vi "Apply Material Theme.vi"(8 "error in":errorcluster, 11 "VI Refnum":refnum<vi>) -> (0 "error out":errorcluster)   [LabVIEW 2021]
doc: "Show this VI and let user define a new path/theme to apply to the VI.\n\n->Will be invoked with Quick Drop as a way to easily change the theme quickly during edit mode\n\n<b>Code Developed By:</b>\nTechnology Service Corporation\nwww.tsc.com/atcs\n\nDeveloper:\nDaniel Coons"
uses:
  Material Theme/Material Theme.lvclass
  user32.dll
panel:
  out "Name of VI":string
  in  "Theme":u16(ring) items=["Light", "Light Medium Contrast", "Light High Contrast", "Dark", "Dark Medium Contrast", "Dark High Contrast"]
  in  "done":bool
  out "header":bool
  in  "Path to theme file":path
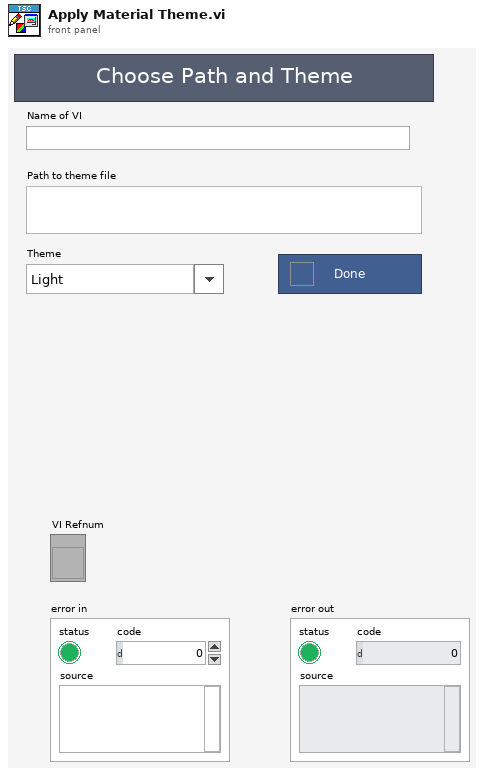
[diagram p1: front panel]
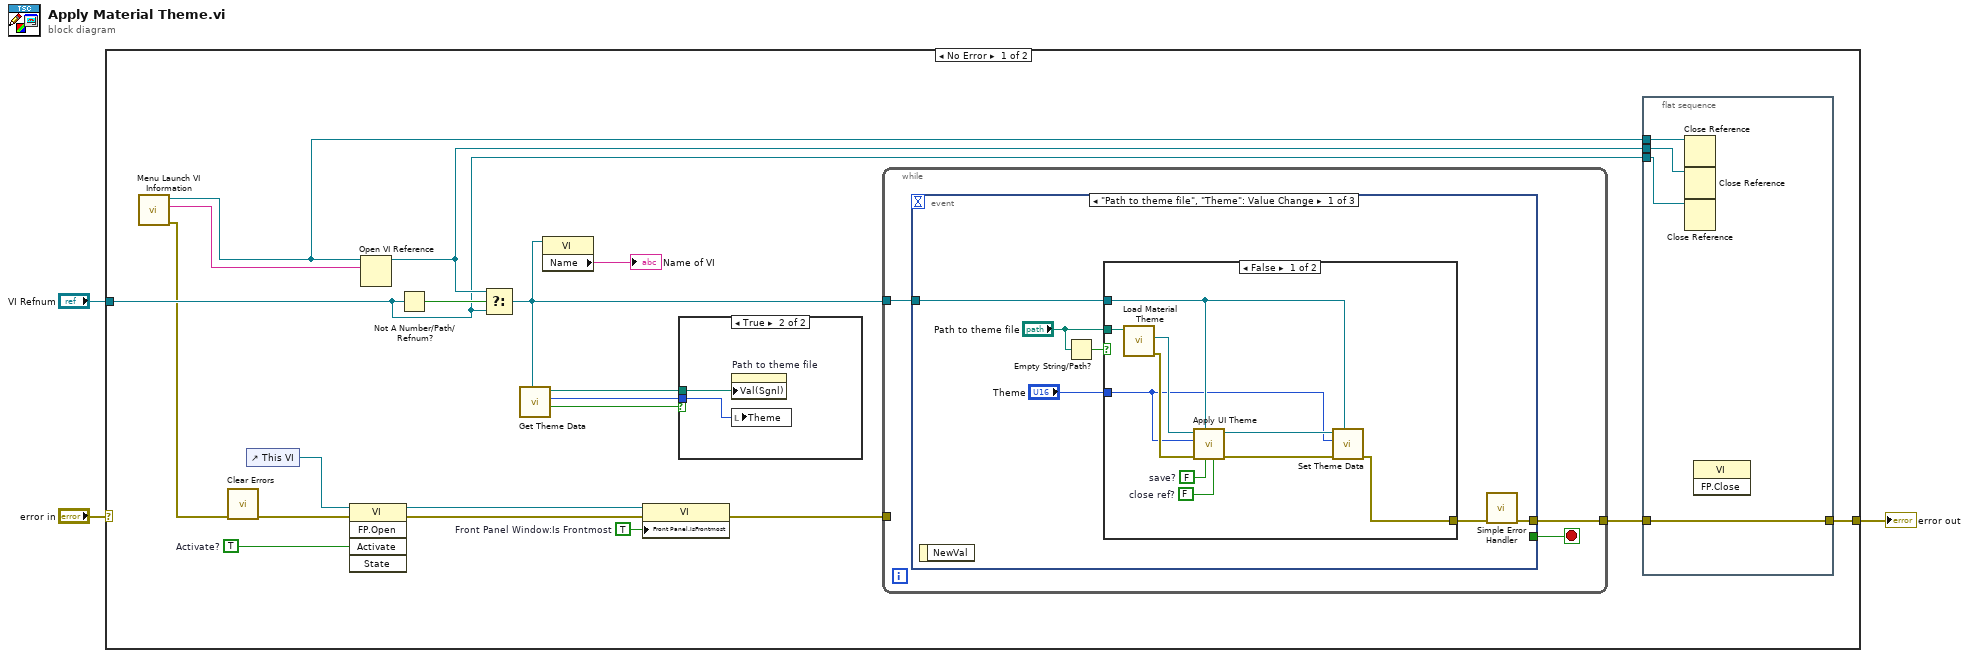
[diagram p0: block diagram]
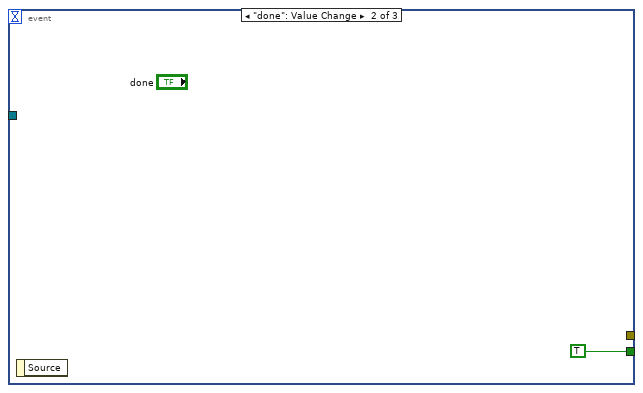
[diagram p4: hidden frame]
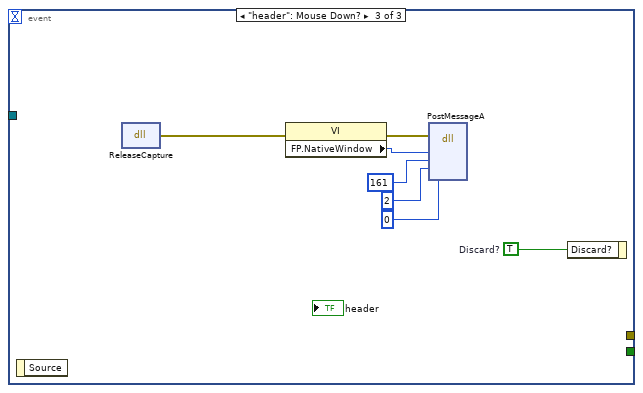
[diagram p5: hidden frame]
diagram:
  n1 = case shown="No Error" "error in" {
    selector: "error in" -> [_ w57]
    tunnel: "VI Refnum" -> [w13 _]
    tunnel: [w20 w57] -> w2
    frame No Error {
      w17 = TRUE  # Front Panel Window:Is Frontmost
      w22 = TRUE  # Activate?
      n2 = call <vilib>:"Menu Launch VI Information.vi"() -> ("error out"=w10:errorcluster, "Menu Launch:VI"=w11:string, "Menu Launch:App"=w12:refnum<vi>)  [unwired: 9 in]
      n3 = call <vilib>:"Clear Errors.vi"("error in (no error)"=w10) -> ("error out"=w8:errorcluster)  [unwired: 5 in, 1 out]
      n4 = control-ref of="This VI"() -> (w9:refnum<vi>)
      n5 = invoke class="VI" method="FP.Open"(reference=w9, error in=w8, "Activate"=w22) -> (reference out=w18:refnum<vi>, error out=w23:errorcluster)  [unwired: 2 in, 3 out]
      n6 = Open VI Reference(application reference (local)=w12, vi path=w11) -> (vi reference=w14:refnum<vi>)  [unwired: 4 in, 1 out]
      n7 = Not A Number/Path/Refnum?(number/path/refnum=w13) -> (NaN/Path/Refnum?=w16:bool)
      n8 = Select(t=w14, s=w16, f=w13) -> (s? t:f=w7:refnum<vi>)
      n9 = call "Get Theme Data.vi"("VI Refnum"=w7) -> ("Found?"=w6:bool, "Theme"=w4:u16, "Theme Path"=w5:path)  [unwired: 7 in, 1 out]
      n10 = property class="VI"(reference=w7) -> ("Name"=→"Name of VI":string)  [unwired: 1 in, 2 out]
      n11 = property class="VI"(reference=w18, error in=w23, "Front Panel.IsFrontmost"=w17) -> (error out=w19:errorcluster)  [unwired: 1 out]
      n12 = case shown="True" w6 {
        tunnel: w5 -> [_ w25]
        tunnel: w4 -> [_ w24]
        frame False {
        }
        frame True {
          n13 = property on="Path to theme file" class="Path"("Val(Sgnl)"=w25) -> ()  [unwired: 2 in, 2 out]
          n14 = local write "Theme"(w24) -> ()
        }
      }
      n15 = while {
        tunnel: w7 -> [w32]
        tunnel: w19 -> [_]
        tunnel: [w31] -> w21
        stop <- w30 stop-if-true
        n16 = event shown="[0] \"Path to theme file\", \"Theme\": Value Change" {
          selector: _ -> [_ _ _]
          dyn-events: _ -> [_ _ _]
          timeout: _ -> [_ _ _]
          tunnel: w32 -> [w38 _ _]
          tunnel: [w36 _ _] -> w31
          tunnel: [_ TRUE _] -> w30
          event "Path to theme file", "Theme": Value Change {
            n17 = event-data() -> ()  [unwired: 1 in, 1 out]
            n18 = Empty String/Path?(string/path="Path to theme file") -> (empty?=w33:bool)
            n19 = case shown="False" w33 {
              tunnel: "Path to theme file" -> [w48 _]
              tunnel: w38 -> [w41 _]
              tunnel: [w42 _] -> w37
              tunnel: "Theme" -> [w39 _]
              frame False {
                w44 = FALSE  # save?
                w45 = FALSE  # close ref?
                n20 = call "Load Material Theme.vi"("file path (use dialog)"=w48) -> ("error out"=w46:errorcluster, "Theme"=w47:refnum<class "Material Theme.lvclass">)  [unwired: 9 in]
                n21 = call "Apply UI Theme.vi"("close ref?"=w45, "save?"=w44, "VI Refnum"=w41, "error in (no error)"=w46, "Theme Mode"=w39, "Material Theme in"=w47) -> ("error out"=w43:errorcluster, "Material Theme out"=w40:refnum<class "Material Theme.lvclass">)  [unwired: 4 in]
                n22 = call "Set Theme Data.vi"("VI Refnum"=w41, "error in"=w43, "Theme"=w39, "Material Theme.lvclass"=w40) -> ("error out"=w42:errorcluster)  [unwired: 7 in]
              }
              frame True {
              }
            }
            n23 = call <vilib>:"Simple Error Handler.vi"("error in (no error)"=w37) -> ("error out"=w36:errorcluster)  [unwired: 4 in, 4 out]
          }
          event "done": Value Change {
            n24 = event-data() -> ()  [unwired: 1 in, 1 out]
          }
          event "header": Mouse Down? {
            w56 = TRUE  # Discard?
            n25 = event-data() -> ()  [unwired: 1 in, 1 out]
            n26 = dll-call lib="user32.dll" fn="ReleaseCapture"() -> (error out=w52:errorcluster)  [unwired: 4 in, 1 out]
            n27 = property class="VI"(error in=w52) -> (error out=w51:errorcluster, "FP.NativeWindow"=w50:u64)  [unwired: 1 in, 1 out]
            n28 = dll-call lib="user32.dll" fn="PostMessageA"(error in=w51, "hWnd"=w50, "Msg"=161, "wParam"=2, "lParam"=0) -> ()  [unwired: 7 in, 2 out]
            n29 = event-data("Discard?"=w56) -> ()  [unwired: 1 in, 1 out]
          }
        }
      }
      n30 = flat-sequence {
        tunnel: w21 -> [w29]
        tunnel: [w29] -> w20
        tunnel: w12 -> [w28]
        tunnel: w14 -> [w27]
        tunnel: w13 -> [w26]
        frame #0 {
          n31 = Close Reference(reference=w28) -> ()  [unwired: 1 in, 1 out]
          n32 = Close Reference(reference=w27) -> ()  [unwired: 1 in, 1 out]
          n33 = Close Reference(reference=w26) -> ()  [unwired: 1 in, 1 out]
          n34 = invoke class="VI" method="FP.Close"() -> ()  [unwired: 3 in, 3 out]
        }
      }
    }
    frame Error {
    }
  }
  "error out" <- w2
